vi "Reset Axis Labels.vi"(8 "error in (no error)":errorcluster, 9 "Root Scene Object out":refnum<vi>, 10 "Actual Transform In":T1, 11 "3D Plot.lvclass in":refnum<class "3D Plot.lvclass">) -> (0 "error out":errorcluster, 1 "Root Scene Object out":refnum<vi>, 2 "Actual Transform Out":T1, 3 "3D Plot.lvclass out":refnum<class "3D Plot.lvclass">)   [LabVIEW 2020, in "3D Plot.lvclass"]
uses:
  <vilib>/Math Plots/3D Math Plots/3D Plot/3D Plot/3D Plot.lvclass
  <vilib>/Math Plots/3D Math Plots/3D Plot/3D Plot/Typedef/Actual Transform.ctl
  <vilib>/Math Plots/3D Math Plots/3D Plot/3D Plot/Typedef/Range Clusters.ctl
  <vilib>/Math Plots/3D Math Plots/3D Plot/3D Plot/3D Plot.lvclass/3D Plot.ctl
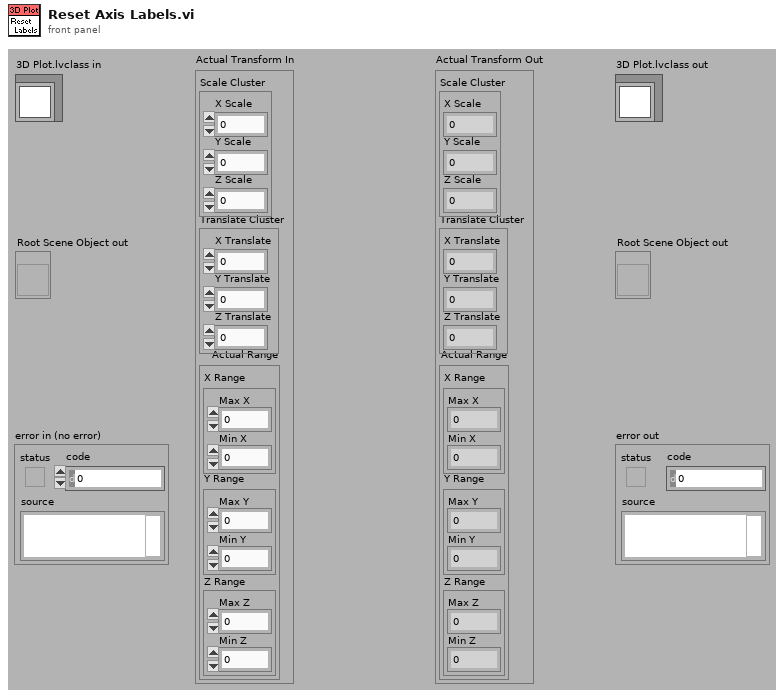
[diagram p1: front panel]
types:
  T1 = typedef "3D Plot.lvclass/Actual Transform.ctl" = cluster{"Scale Cluster":cluster{"X Scale":sgl, "Y Scale":sgl, "Z Scale":sgl}, "Translate Cluster":cluster{"X Translate":sgl, "Y Translate":sgl, "Z Translate":sgl}, "Actual Range":T2}
  T2 = typedef "3D Plot.lvclass/Range Clusters.ctl" = cluster{"X Range":cluster{"Max X":sgl, "Min X":sgl}, "Y Range":cluster{"Max Y":sgl, "Min Y":sgl}, "Z Range":cluster{"Max Z":sgl, "Min Z":sgl}}
  T3 = enum16{"X", "Y", "Z", "X Opposite", "Y Opposite", "Z Opposite"}
  T4 = typedef "3D Plot.lvclass/Tick Array Cluster.ctl" = cluster{"X Tick Array":T5, "Y Tick Array":T5, "Z Tick Array":T5}
  T5 = typedef "3D Plot.lvclass/Tick Array.ctl" = cluster{"Label":bool, "Show Tick":bool, "Show Line":bool, "Value Numeric":sgl, "Value String":string}[]
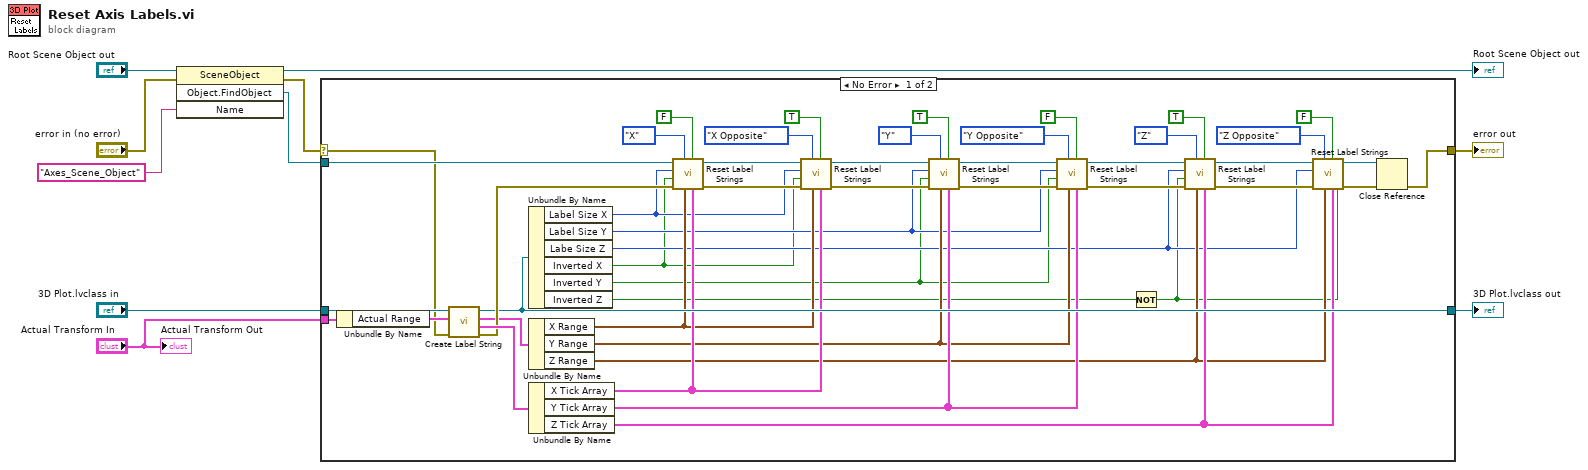
[diagram p0: block diagram]
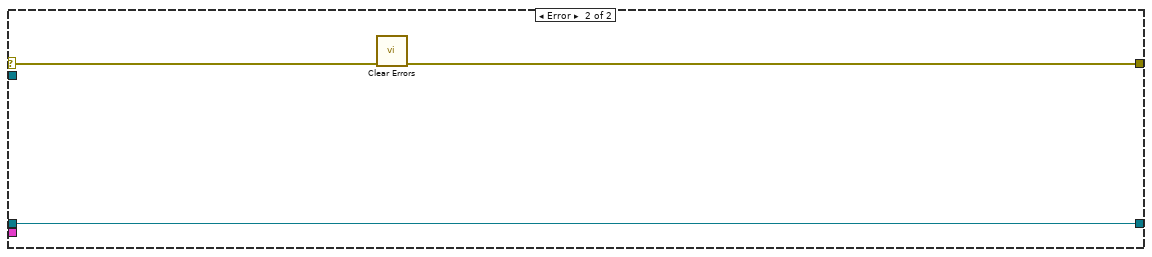
[diagram p2: hidden frame]
diagram:
  n1 = invoke class="SceneObject" method="Object.FindObject"(reference="Root Scene Object out", error in="error in (no error)", "Name"="Axes_Scene_Object") -> (reference out=→"Root Scene Object out":refnum<vi>, error out=w2:errorcluster, "FindObject"=w9:refnum<vi>)  [unwired: 1 in, 1 out]
  n2 = case shown="No Error" w2 {
    selector: w2 -> [w47 w58]
    tunnel: [w18 w59] -> w8
    tunnel: w9 -> [w54 _]
    tunnel: "3D Plot.lvclass in" -> [w57 w60]
    tunnel: "Actual Transform In" -> [w56 _]
    tunnel: [w46 w60] -> w5
    frame No Error {
      n3 = Unbundle By Name(w56) -> ("Actual Range"=w55:T2)
      n4 = call <vilib>:"Create Label String.vi"("error in (no error)"=w47, "Actual Range In"=w55, "3D Plot.lvclass in"=w57) -> ("error out"=w48:errorcluster, "Label Cluster"=w53:T4, "Actual Range Out"=w39:T2, "3D Plot.lvclass out"=w46:refnum<class "3D Plot.lvclass">)  [unwired: 1 in, 4 out]
      n5 = Unbundle By Name(w46) -> ("Label Size X"=w25:u16, "Label Size Y"=w24:u16, "Labe Size Z"=w23:u16, "Inverted X"=w22:bool, "Inverted Y"=w20:bool, "Inverted Z"=w21:bool)
      n6 = Unbundle By Name(w39) -> ("X Range"=w33:cluster{"Max X":sgl, "Min X":sgl}, "Y Range"=w32:cluster{"Max Y":sgl, "Min Y":sgl}, "Z Range"=w34:cluster{"Max Z":sgl, "Min Z":sgl})
      n7 = Unbundle By Name(w53) -> ("X Tick Array"=w38:T5, "Y Tick Array"=w37:T5, "Z Tick Array"=w36:T5)
      n8 = call <vilib>:"Reset Label Strings.vi"("Tick Array"=w38, "Right justified"=FALSE, "Range"=w33, "Which Axis?"=T3."X", "error in (no error)"=w48, "Inverted?"=w22, "Size"=w25, "Axis Scene Object in"=w54) -> ("error out"=w50:errorcluster, "Axis Scene Object out"=w51:refnum<vi>)  [unwired: 2 in]
      n9 = call <vilib>:"Reset Label Strings.vi"("Tick Array"=w38, "Right justified"=TRUE, "Range"=w33, "Which Axis?"=T3."X Opposite", "error in (no error)"=w50, "Inverted?"=w22, "Size"=w25, "Axis Scene Object in"=w51) -> ("error out"=w49:errorcluster, "Axis Scene Object out"=w52:refnum<vi>)  [unwired: 2 in]
      n10 = call <vilib>:"Reset Label Strings.vi"("Tick Array"=w37, "Right justified"=TRUE, "Range"=w32, "Which Axis?"=T3."Y", "error in (no error)"=w49, "Inverted?"=w20, "Size"=w24, "Axis Scene Object in"=w52) -> ("error out"=w42:errorcluster, "Axis Scene Object out"=w45:refnum<vi>)  [unwired: 2 in]
      n11 = call <vilib>:"Reset Label Strings.vi"("Tick Array"=w37, "Right justified"=FALSE, "Range"=w32, "Which Axis?"=T3."Y Opposite", "error in (no error)"=w42, "Inverted?"=w20, "Size"=w24, "Axis Scene Object in"=w45) -> ("error out"=w41:errorcluster, "Axis Scene Object out"=w43:refnum<vi>)  [unwired: 2 in]
      n12 = Not(x=w21) -> (.not. x?=w17:bool)
      n13 = call <vilib>:"Reset Label Strings.vi"("Tick Array"=w36, "Right justified"=TRUE, "Range"=w34, "Which Axis?"=T3."Z", "error in (no error)"=w41, "Inverted?"=w17, "Size"=w23, "Axis Scene Object in"=w43) -> ("error out"=w40:errorcluster, "Axis Scene Object out"=w44:refnum<vi>)  [unwired: 2 in]
      n14 = call <vilib>:"Reset Label Strings.vi"("Tick Array"=w36, "Right justified"=FALSE, "Range"=w34, "Which Axis?"=T3."Z Opposite", "error in (no error)"=w40, "Inverted?"=w17, "Size"=w23, "Axis Scene Object in"=w44) -> ("error out"=w19:errorcluster, "Axis Scene Object out"=w35:refnum<vi>)  [unwired: 2 in]
      n15 = Close Reference(reference=w35, error in (no error)=w19) -> (error out=w18:errorcluster)
    }
    frame Error {
      n16 = call <vilib>:"Clear Errors.vi"("error in (no error)"=w58) -> ("error out"=w59:errorcluster)  [unwired: 5 in, 1 out]
    }
  }
  "error out" <- w8
  "3D Plot.lvclass out" <- w5
  "Actual Transform Out" <- "Actual Transform In"
